vi "이벤트 예제.vi"() -> ()   [LabVIEW 2014]
panel:
  out "웨이브폼 차트":dbl(graph)
  in  "Stop":bool
  in  "Plot":bool
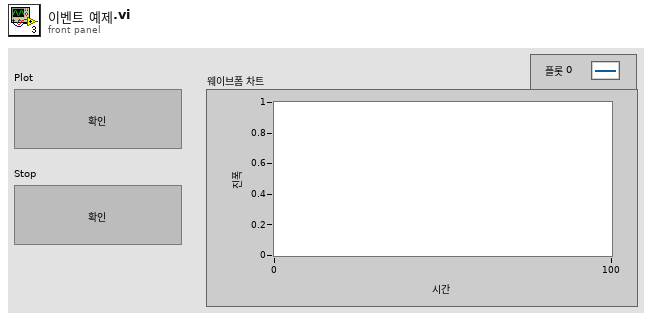
[diagram p1: front panel]
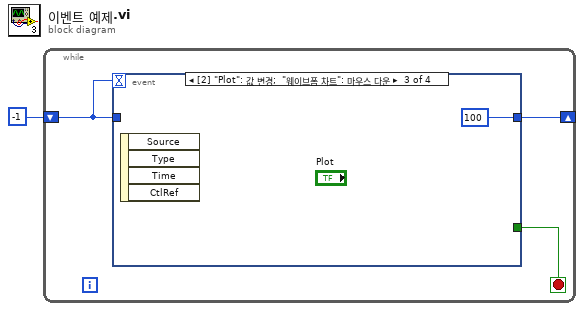
[diagram p0: block diagram]
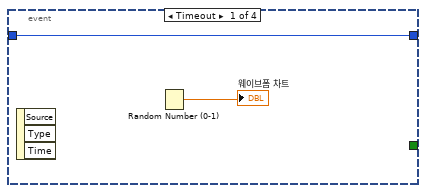
[diagram p2: hidden frame]
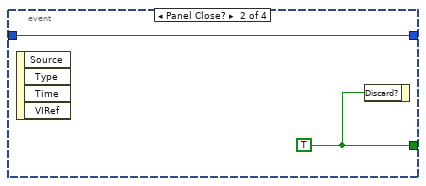
[diagram p3: hidden frame]
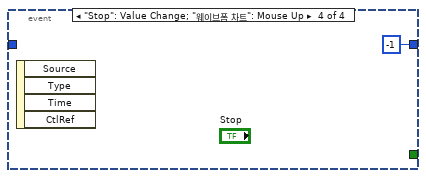
[diagram p4: hidden frame]
diagram:
  n1 = while {
    shift-right: [w2] -> _
    shift-left: -1 -> [w3]
    stop <- w4 stop-if-true
    n2 = event shown="[2] \"Plot\": 값 변경;  \"웨이브폼 차트\": 마우스 다운" {
      selector: _ -> [_ _ _ _]
      dyn-events: _ -> [_ _ _ _]
      timeout: w3 -> [_ _ _ _]
      tunnel: [_ w7 _ _] -> w4
      tunnel: w3 -> [w6 w8 _ _]
      tunnel: [w6 w8 100 -1] -> w2
      event Timeout {
        n3 = event-data() -> ()  [unwired: 1 in, 3 out]
        n4 = Random Number (0-1)() -> (number: 0 to 1=→"웨이브폼 차트":dbl)
      }
      event Panel Close? {
        w7 = TRUE
        n5 = event-data() -> ()  [unwired: 1 in, 4 out]
        n6 = event-data("Discard?"=w7) -> ()  [unwired: 1 in, 1 out]
      }
      event "Plot": Value Change; "웨이브폼 차트": Mouse Down {
        n7 = event-data() -> ()  [unwired: 1 in, 4 out]
      }
      event "Stop": Value Change; "웨이브폼 차트": Mouse Up {
        n8 = event-data() -> ()  [unwired: 1 in, 4 out]
      }
    }
  }
